vi "Autosize Columns (Table).vi"(8 "error in (no error)":errorcluster, 11 "table":refnum<vi>) -> (0 "error out":errorcluster)   [LabVIEW 2023, in "UI Helpers.lvlib"]
uses:
  UI Helpers.lvlib
  <vilib>/Utility/miscctls.llb/LVRowAndColumnTypeDef.ctl
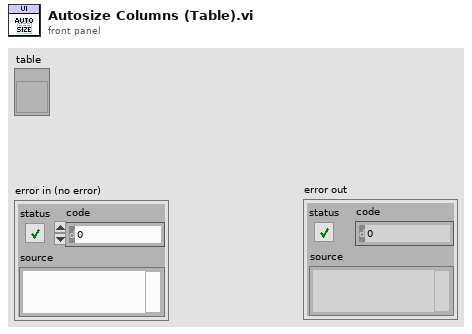
[diagram p1: front panel]
types:
  T1 = enum16{"User-specified Font", "Application Font", "System Font", "Dialog Font"}
  T2 = cluster{"Font Name:":string, "Size":i16, "Strikeout?":bool, "Italic?":bool, "Underline?":bool, "Outline?":bool, "Shadow?":bool, "Bold?":bool}
  T3 = typedef "LVRowAndColumnTypeDef.ctl" = cluster{"Row":i32, "Column":i32}
  T4 = cluster{"left":i16, "top":i16, "right":i16, "bottom":i16}
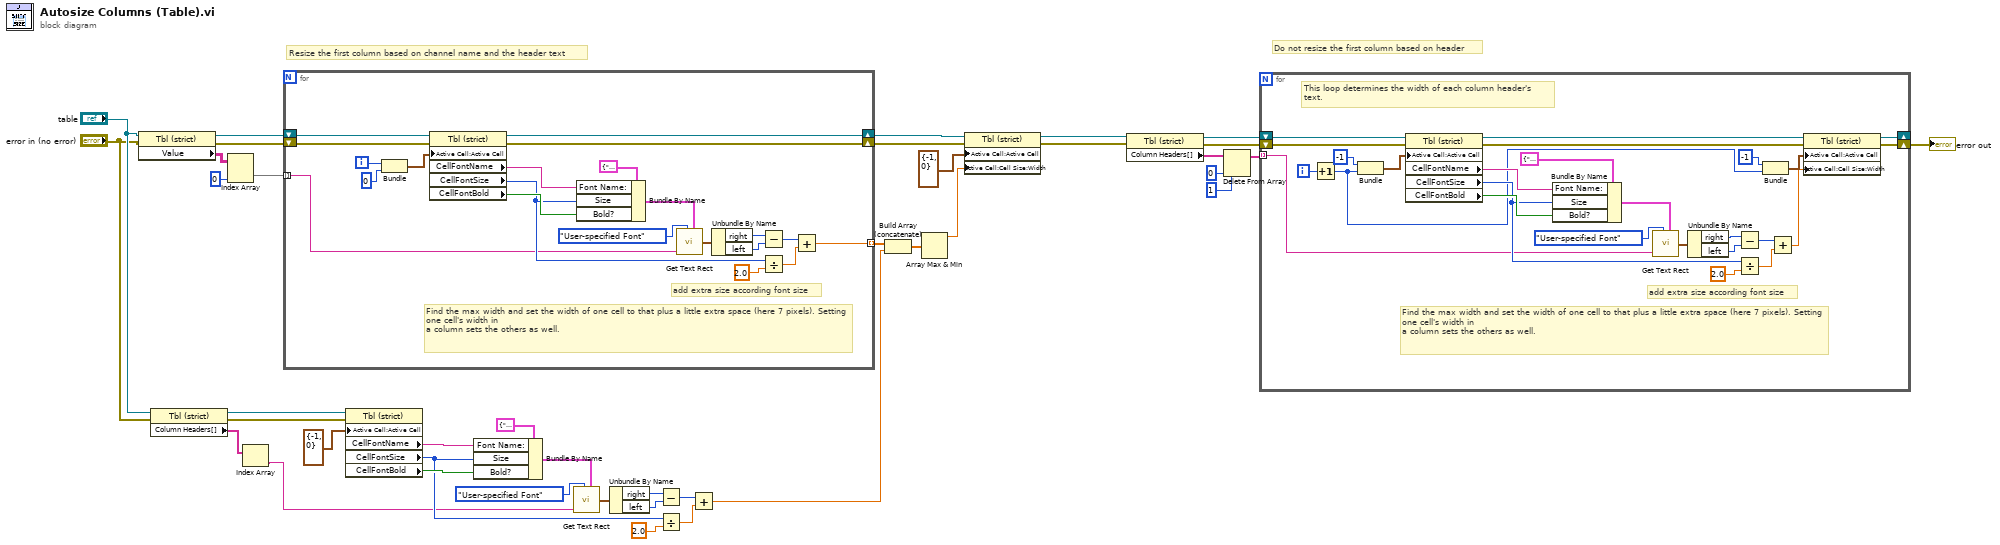
[diagram p0: block diagram]
diagram:
  # "Resize the first column based on channel name and the header text"
  # "Do not resize the first column based on header"
  n1 = property on="Property Node" class="Tbl (strict)"(reference="table", error in="error in (no error)") -> (reference out=w35:refnum<vi>, error out=w34:errorcluster, "Value"=w37:string[][])
  n2 = property on="Property Node" class="Tbl (strict)"(reference="table", error in="error in (no error)") -> (reference out=w19:refnum<vi>, error out=w18:errorcluster, "Column Headers[]"=w20:string[])
  n3 = Index Array(array=w37, index (col)=0 ("disabled index (col)")) -> (element=w33:string[])  [unwired: 1 in]
  n4 = Index Array(array=w20) -> (element=w1:string)  [unwired: 1 in]
  n5 = for {
    shift-right: [w42] -> w29
    shift-left: w35 -> [w58]
    shift-right: [w41] -> w30
    shift-left: w34 -> [w59]
    tunnel: w33 -> [w46] mode=indexing
    tunnel: [w43] -> w4 mode=indexing
    i -> [w44]
    # "add extra size according font size"
    # "Find the max width and set the width of one cell to that plus a little extra space (here 7 pixels). Setting one cell's width in\na column sets the others as well."
    n6 = Bundle(w44, 0) -> (w54:cluster{i32, i32})  [unwired: 1 in]
    n7 = property on="Property Node" class="Tbl (strict)"(reference=w58, error in=w59, "Active Cell:Active Cell"=w54) -> (reference out=w42:refnum<vi>, error out=w41:errorcluster, "CellFontName"=w53:string, "CellFontSize"=w48:u32, "CellFontBold"=w52:bool)
    n8 = Bundle By Name(cluster=T2 {"Font Name:"="", "Size"=0, "Strikeout?"=FALSE, "Italic?"=FALSE, "Underline?"=FALSE, "Outline?"=FALSE, "Shadow?"=FALSE, "Bold?"=FALSE} ("[user-specified font]"), "Font Name:"=w53, "Size"=w48, "Bold?"=w52) -> (w50:T2)
    n9 = call <vilib>:"Get Text Rect.vi"("desired font(Application)"=T1."User-specified Font", "text"=w46, "[user-specified font]"=w50) -> ("rect"=w57:T4)  [unwired: 6 in]
    n10 = Unbundle By Name(w57) -> ("right"=w56:i16, "left"=w55:i16)
    n11 = Subtract(x=w56, y=w55) -> (x-y=w47:i16)
    n12 = Divide(x=w48, y=sgl 2.0) -> (x/y=w60:sgl)
    n13 = Add(x=w47, y=w60) -> (x+y=w43:sgl)
  }
  n14 = property on="Property Node" class="Tbl (strict)"(reference=w19, error in=w18, "Active Cell:Active Cell"=T3 {"Row"=-1, "Column"=0}) -> ("CellFontName"=w7:string, "CellFontSize"=w5:u32, "CellFontBold"=w6:bool)  [unwired: 2 out]
  n15 = Bundle By Name(cluster=T2 {"Font Name:"="", "Size"=0, "Strikeout?"=FALSE, "Italic?"=FALSE, "Underline?"=FALSE, "Outline?"=FALSE, "Shadow?"=FALSE, "Bold?"=FALSE} ("[user-specified font]"), "Font Name:"=w7, "Size"=w5, "Bold?"=w6) -> (w10:T2)
  n16 = call <vilib>:"Get Text Rect.vi"("desired font(Application)"=T1."User-specified Font", "text"=w1, "[user-specified font]"=w10) -> ("rect"=w14:T4)  [unwired: 6 in]
  n17 = Unbundle By Name(w14) -> ("right"=w13:i16, "left"=w12:i16)
  n18 = Subtract(x=w13, y=w12) -> (x-y=w8:i16)
  n19 = Divide(x=w5, y=sgl 2.0) -> (x/y=w15:sgl)
  n20 = Add(x=w8, y=w15) -> (x+y=w3:sgl)
  n21 = Build Array (concatenate)(w4, w3) -> (w2:sgl[])
  n22 = Array Max & Min(array=w2) -> (max value=w28:sgl)  [unwired: 3 out]
  n23 = property on="Property Node" class="Tbl (strict)"(reference=w29, error in=w30, "Active Cell:Active Cell"=T3 {"Row"=-1, "Column"=0}, "Active Cell:Cell Size:Width"=w28) -> (reference out=w27:refnum<vi>, error out=w26:errorcluster)
  n24 = property on="Property Node" class="Tbl (strict)"(reference=w27, error in=w26) -> (reference out=w39:refnum<vi>, error out=w40:errorcluster, "Column Headers[]"=w24:string[])
  n25 = Delete From Array(array=w24, length=1, index=0) -> (array with subset deleted=w23:string[])  [unwired: 1 out]
  n26 = for {
    shift-right: [w77] -> _
    shift-left: w39 -> [w82]
    shift-right: [w81] -> w38
    shift-left: w40 -> [w83]
    tunnel: w23 -> [w64] mode=indexing
    i -> [w63]
    # "This loop determines the width of each column header's\ntext."
    # "add extra size according font size"
    # "Find the max width and set the width of one cell to that plus a little extra space (here 7 pixels). Setting one cell's width in\na column sets the others as well."
    n27 = Increment(x=w63) -> (x+1=w62:i32)
    n28 = Bundle(-1, w62) -> (w73:cluster{i32, i32})  [unwired: 1 in]
    n29 = property on="Property Node" class="Tbl (strict)"(reference=w82, error in=w83, "Active Cell:Active Cell"=w73) -> (reference out=w80:refnum<vi>, error out=w79:errorcluster, "CellFontName"=w72:string, "CellFontSize"=w66:u32, "CellFontBold"=w71:bool)
    n30 = Bundle By Name(cluster=T2 {"Font Name:"="", "Size"=0, "Strikeout?"=FALSE, "Italic?"=FALSE, "Underline?"=FALSE, "Outline?"=FALSE, "Shadow?"=FALSE, "Bold?"=FALSE} ("[user-specified font]"), "Font Name:"=w72, "Size"=w66, "Bold?"=w71) -> (w69:T2)
    n31 = call <vilib>:"Get Text Rect.vi"("desired font(Application)"=T1."User-specified Font", "text"=w64, "[user-specified font]"=w69) -> ("rect"=w76:T4)  [unwired: 6 in]
    n32 = Unbundle By Name(w76) -> ("right"=w75:i16, "left"=w74:i16)
    n33 = Subtract(x=w75, y=w74) -> (x-y=w65:i16)
    n34 = Divide(x=w66, y=sgl 2.0) -> (x/y=w84:sgl)
    n35 = Bundle(-1, w62) -> (w86:cluster{i32, i32})  [unwired: 1 in]
    n36 = Add(x=w65, y=w84) -> (x+y=w78:sgl)
    n37 = property on="Property Node" class="Tbl (strict)"(reference=w80, error in=w79, "Active Cell:Active Cell"=w86, "Active Cell:Cell Size:Width"=w78) -> (reference out=w77:refnum<vi>, error out=w81:errorcluster)
  }
  "error out" <- w38
